vi "Battery Model Loop.vi"() -> ()   [LabVIEW 2014]
uses:
  Current Voltage Sample.ctl
  <vilib>/Analysis/6fits.llb/Curve Fitting Criteria.ctl
  <vilib>/FPGAPlugInAG/sbRIO-9626/niLvFpga_Open_sbRIO-9626.vi
  Global Data.vi
  <vilib>/Utility/error.llb/Error Cluster From Error Code.vi
  <vilib>/rvi/errors/niLvFpgaAdjustHostInterfaceError.vi
  <vilib>/FPGAPlugInAG/sbRIO-9626/niLvFpga_Close_sbRIO-9626.vi
  <vilib>/rvi/interface/nirviOpenFPGA/nirviOpenFPGA.xnode
  FPGA Bitfiles/Latest.lvbitx
  <vilib>/rvi/interface/nirviReadWriteControl/nirviReadWriteControl.xnode
  <vilib>/rvi/interface/nirviCloseFPGA/nirviCloseFPGA.xnode
  NiFpgaLv.dll
  <vilib>/Analysis/NI_AALPro.lvlib
panel:
  out "IBatteryMaxTarget":dbl
  out "r^2":dbl
  out "intercept (V)":dbl
  out "slope (V / A)":dbl
  out "tICurrentAccumulated":dbl
  in  "bResetCurrentAccumulator":bool
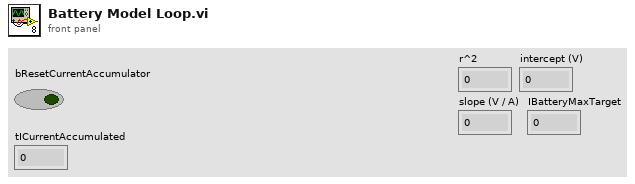
[diagram p1: front panel]
types:
  T1 = typedef "Current Voltage Sample.ctl" = cluster{"IAverage":dbl, "VCellMin":dbl, "tSampleDuration":u32}
  T2 = typedef "BMS Telemetry.ctl" = cluster{"bBMSIgnition":bool, "bBMSChargerMains":bool, "bBMSFastCharge":bool, "bBMSChargerEnabled":bool, "eBMSCarState":enum16{"Off", "On, Not Charging", "Charging", "Charging Finished", "Charging Error"}, "eBMSChargingState":enum16{"Disconnected", "Pre-charging", "Main Charging", "Balancing", "Charging Finished OK", "Charging Error"}, "tBMSChargeStage":u16, "eBMSLastChargeError":enum16{"No Error", "No Cell Communication", "No Cell Communication - Non CAN Charger", "Maximum charging stage duration expired", "Cell Communication Lost during Charge", "Cannot set balancing voltage", "Cell temps too high", "No Comms so can't determine temp", "# of Cells Mismatch", "Cells Overvoltage", "Cell Protection Event occured."}, "NBMSNumCells":u8, "bBMSUnderVProtection":bool, "bBMSOverVProtection":bool, "bBMSOverTProtection":bool, "bBMSLeakageProtection":bool, "bBMSNoCellCommsError":bool, "bBMSLowVReduction":bool, "bBMSHighTReduction":bool, "VCellMin":dbl, "VCellMax":dbl, "VCellMean":dbl, "VTotal":dbl, "TCellMin":dbl, "TCellMax":dbl, "TCellMean":dbl, "VCells":cluster{"[51]":dbl, "[52]":dbl, "[53]":dbl, "[54]":dbl, "[55]":dbl, "[56]":dbl, "[57]":dbl, "[58]":dbl, "[59]":dbl, "[60]":dbl, "[61]":dbl, "[62]":dbl, "[63]":dbl, "[64]":dbl, "[65]":dbl, "[66]":dbl, "[67]":dbl, "[34]":dbl, "[35]":dbl, "[36]":dbl, "[37]":dbl, "[38]":dbl, "[39]":dbl, "[40]":dbl, "[41]":dbl, "[42]":dbl, "[43]":dbl, "[44]":dbl, "[45]":dbl, "[46]":dbl, "[47]":dbl, "[48]":dbl, "[49]":dbl, "[50]":dbl, "[17]":dbl, "[18]":dbl, "[19]":dbl, "[20]":dbl, "[21]":dbl, "[22]":dbl, "[23]":dbl, "[24]":dbl, "[25]":dbl, "[26]":dbl, "[27]":dbl, "[28]":dbl, "[29]":dbl, "[30]":dbl, "[31]":dbl, "[32]":dbl, "[33]":dbl, "[0]":dbl, "[1]":dbl, "[2]":dbl, "[3]":dbl, "[4]":dbl, "[5]":dbl, "[6]":dbl, "[7]":dbl, "[8]":dbl, "[9]":dbl, "[10]":dbl, "[11]":dbl, "[12]":dbl, "[13]":dbl, "[14]":dbl, "[15]":dbl, "[16]":dbl}, "TCells":cluster{"[55]":dbl, "[56]":dbl, "[57]":dbl, "[58]":dbl, "[59]":dbl, "[60]":dbl, "[61]":dbl, "[62]":dbl, "[63]":dbl, "[64]":dbl, "[65]":dbl, "[66]":dbl, "[67]":dbl, "[68]":dbl, "[69]":dbl, "[70]":dbl, "[17]":dbl, "[38]":dbl, "[39]":dbl, "[40]":dbl, "[41]":dbl, "[42]":dbl, "[43]":dbl, "[44]":dbl, "[45]":dbl, "[46]":dbl, "[47]":dbl, "[48]":dbl, "[49]":dbl, "[50]":dbl, "[51]":dbl, "[52]":dbl, "[53]":dbl, "[54]":dbl, "[21]":dbl, "[22]":dbl, "[23]":dbl, "[24]":dbl, "[25]":dbl, "[26]":dbl, "[27]":dbl, "[28]":dbl, "[29]":dbl, "[30]":dbl, "[31]":dbl, "[32]":dbl, "[33]":dbl, "[34]":dbl, "[35]":dbl, "[36]":dbl, "[37]":dbl, "[0]":dbl, "[1]":dbl, "[2]":dbl, "[3]":dbl, "[4]":dbl, "[5]":dbl, "[6]":dbl, "[7]":dbl, "[8]":dbl, "[9]":dbl, "[10]":dbl, "[11]":dbl, "[12]":dbl, "[13]":dbl, "[14]":dbl, "[15]":dbl, "[16]":dbl}, "bChargerConnected":bool, "VChargerSetpoint":dbl, "IChargerSetpoint":dbl, "VChargerActual":dbl, "IChargerActual":dbl, "BCells":cluster{"[51]":dbl, "[52]":dbl, "[53]":dbl, "[54]":dbl, "[55]":dbl, "[56]":dbl, "[57]":dbl, "[58]":dbl, "[59]":dbl, "[60]":dbl, "[61]":dbl, "[62]":dbl, "[63]":dbl, "[64]":dbl, "[65]":dbl, "[66]":dbl, "[67]":dbl, "[34]":dbl, "[35]":dbl, "[36]":dbl, "[37]":dbl, "[38]":dbl, "[39]":dbl, "[40]":dbl, "[41]":dbl, "[42]":dbl, "[43]":dbl, "[44]":dbl, "[45]":dbl, "[46]":dbl, "[47]":dbl, "[48]":dbl, "[49]":dbl, "[50]":dbl, "[17]":dbl, "[18]":dbl, "[19]":dbl, "[20]":dbl, "[21]":dbl, "[22]":dbl, "[23]":dbl, "[24]":dbl, "[25]":dbl, "[26]":dbl, "[27]":dbl, "[28]":dbl, "[29]":dbl, "[30]":dbl, "[31]":dbl, "[32]":dbl, "[33]":dbl, "[0]":dbl, "[1]":dbl, "[2]":dbl, "[3]":dbl, "[4]":dbl, "[5]":dbl, "[6]":dbl, "[7]":dbl, "[8]":dbl, "[9]":dbl, "[10]":dbl, "[11]":dbl, "[12]":dbl, "[13]":dbl, "[14]":dbl, "[15]":dbl, "[16]":dbl}, "bNewVCellMinSample":bool}
  T3 = typedef "NI_AALPro.lvlib/Curve Fitting Criteria.ctl" = u16
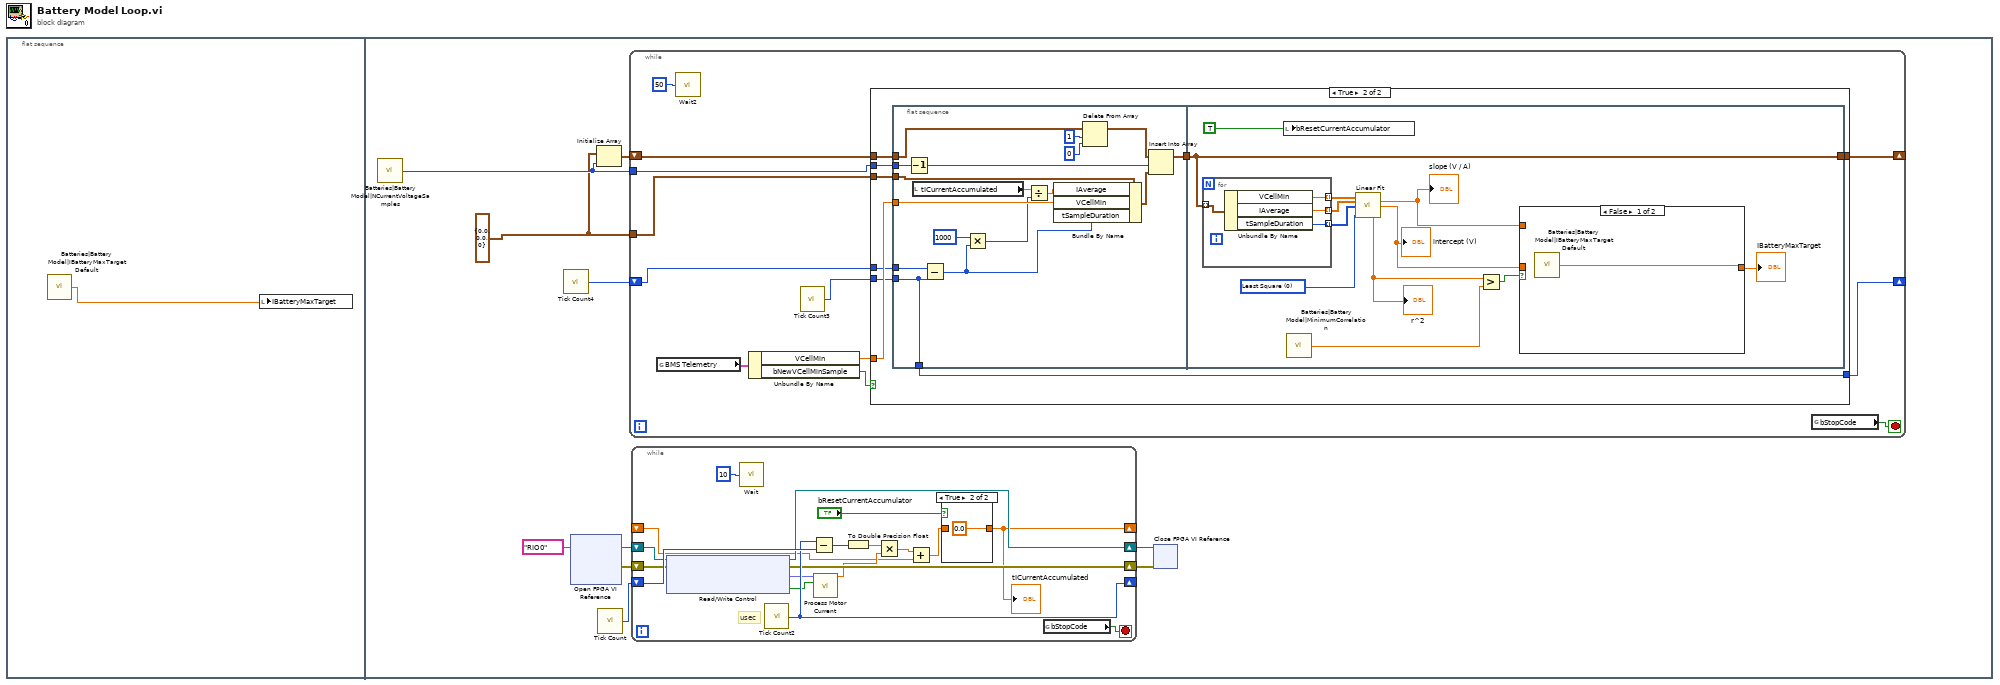
[diagram p0: block diagram]
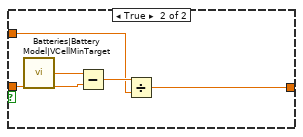
[diagram p4: hidden frame]
diagram:
  n1 = flat-sequence {
    frame #0 {
      n2 = call "Batteries|Battery Model|IBatteryMaxTargetDefault"() -> ("Value"=w1:sgl)
      n3 = local write "IBatteryMaxTarget"(w1) -> ()
    }
    frame #1 {
      w3 = T1 {"IAverage"=0.0, "VCellMin"=0.0, "tSampleDuration"=0} ("Current Voltage Sample")
      n4 = call "Batteries|Battery Model|NCurrentVoltageSamples"() -> ("Value"=w10:i32)
      n5 = call "Tick Count4"() -> ("Tick Count(mSec)"=w4:u32)
      n6 = xnode "Open FPGA VI Reference"("resource name"=tag "RIO0") -> ("FPGA VI Reference Out"=w8:refnum<k20>, "error out"=w7:errorcluster)  [unwired: 1 in]
      n7 = Initialize Array(w3, w10) -> (w11:T1[])
      n8 = call "Tick Count"() -> ("Tick Count(uSec)"=w9:u32)
      n9 = while {
        shift-right: [w39] -> _
        shift-left: w11 -> [w40]
        tunnel: w10 -> [w38]
        tunnel: w3 -> [w37]
        shift-right: [w32] -> _
        shift-left: w4 -> [w34]
        stop <- w43 stop-if-true
        n10 = global read "Global Data.vi" "BMS Telemetry"() -> (w42:T2)
        n11 = call "Wait2"("Count(mSec)"=u32 50) -> ()  [unwired: 1 out]
        n12 = Unbundle By Name(w42) -> ("VCellMin"=w36:dbl, "bNewVCellMinSample"=w41:bool)
        n13 = call "Tick Count3"() -> ("Tick Count(mSec)"=w33:u32)
        n14 = case shown="True" w41 {
          tunnel: w40 -> [w45 w54]
          tunnel: [w45 w50] -> w39
          tunnel: w38 -> [_ w53]
          tunnel: w37 -> [_ w52]
          tunnel: w36 -> [_ w51]
          tunnel: w34 -> [w44 w48]
          tunnel: w33 -> [_ w47]
          tunnel: [w44 w46] -> w32
          frame False {
          }
          frame True {
            n15 = flat-sequence {
              tunnel: w54 -> [w71]
              tunnel: w53 -> [w67]
              tunnel: w52 -> [w65]
              tunnel: w51 -> [w63]
              tunnel: [w62] -> w49
              tunnel: w48 -> [w61]
              tunnel: w47 -> [w60]
              tunnel: [w60] -> w46
              tunnel: [w82] -> w50
              tunnel: w49 -> [w82]
              frame #0 {
                n16 = Decrement(x=w67) -> (x-1=w66:i32)
                n17 = local read "tICurrentAccumulated"() -> (w58:dbl)
                n18 = Subtract(x=w61, y=w60) -> (x-y=w57:u32)
                n19 = Multiply(x=u32 1000, y=w57) -> (x*y=w55:u32)
                n20 = Divide(x=w58, y=w55) -> (x/y=w59:dbl)
                n21 = Bundle By Name(cluster=w65, "IAverage"=w59, "VCellMin"=w63, "tSampleDuration"=w57) -> (w64:T1)
                n22 = Delete From Array(array=w71, length=1, index=0) -> (array with subset deleted=w68:T1[])  [unwired: 1 out]
                n23 = Insert Into Array(array=w68, index=w66, new element=w64) -> (w62:T1[])
              }
              frame #1 {
                w78 = T3 0 items=["Least Square", "Least Absolute Residual", "Bisquare"] ("method")
                n24 = for {
                  tunnel: w82 -> [w93] mode=indexing
                  tunnel: [w92] -> w81 mode=indexing
                  tunnel: [w91] -> w80 mode=indexing
                  tunnel: [w90] -> w79 mode=indexing
                  n25 = Unbundle By Name(w93) -> ("VCellMin"=w92:dbl, "IAverage"=w91:dbl, "tSampleDuration"=w90:u32)
                }
                n26 = local write "bResetCurrentAccumulator"(TRUE ("bResetCurrentAccumulator")) -> ()
                n27 = call "Batteries|Battery Model|MinimumCorrelation"() -> ("Value"=w76:sgl)
                n28 = call <vilib>:"Linear Fit.vi"("Y"=w81, "X"=w80, "Weight"=w79, "method"=w78) -> ("slope"=w73:dbl, "intercept"=w74:dbl, "residue"=w77:dbl)  [unwired: 7 in, 2 out]
                "slope (V / A)" <- w73
                "intercept (V)" <- w74
                "r^2" <- w77
                n29 = Greater?(x=w77, y=w76) -> (0:w75:bool)
                n30 = case shown="False" w75 {
                  tunnel: w74 -> [_ w88]
                  tunnel: w73 -> [_ w86]
                  tunnel: [w84 w85] -> w72
                  frame False {
                    n31 = call "Batteries|Battery Model|IBatteryMaxTargetDefault"() -> ("Value"=w84:sgl)
                  }
                  frame True {
                    n32 = call "Batteries|Battery Model|VCellMinTarget"() -> ("Value"=w89:sgl)
                    n33 = Subtract(x=w89, y=w88) -> (x-y=w87:dbl)
                    n34 = Divide(x=w87, y=w86) -> (x/y=w85:dbl)
                  }
                }
                "IBatteryMaxTarget" <- w72
              }
            }
          }
        }
        n35 = global read "Global Data.vi" "bStopCode"() -> (w43:bool)
      }
      n36 = while {
        shift-right: [w26] -> _
        shift-left: w9 -> [w27]
        shift-right: [w21] -> w6
        shift-left: w8 -> [w25]
        shift-right: [w20] -> w5
        shift-left: w7 -> [w24]
        shift-right: [w12] -> _
        shift-left: _ -> [w15]
        stop <- w28 stop-if-true
        # "usec"
        n37 = xnode "Read/Write Control"("FPGA VI Reference In"=w25, "error in"=w24) -> ("FPGA VI Reference Out"=w21:refnum<k20>, "error out"=w20:errorcluster, "IHighCurrent"=w23:fxp<+/-,19,15>, "bHighCurrentOK"=w22:bool)
        n38 = call "Wait"("Count(mSec)"=u32 10) -> ()  [unwired: 1 out]
        n39 = call "Tick Count2"() -> ("Tick Count(uSec)"=w26:u32)
        n40 = Subtract(x=w26, y=w27) -> (x-y=w17:u32)
        n41 = call "Process Motor Current.vi"("bHighCurrentOK"=w22, "IHighCurrent"=w23) -> ("IMotor"=w19:dbl)  [unwired: 8 in, 1 out]
        n42 = To Double Precision Float(number=w17) -> (double precision float=w18:dbl)
        n43 = Multiply(x=w18, y=w19) -> (x*y=w16:dbl)
        n44 = Add(x=w16, y=w15) -> (x+y=w14:dbl)
        n45 = case shown="True" "bResetCurrentAccumulator" {
          tunnel: w14 -> [w30 _]
          tunnel: [w30 0.0] -> w12
          frame False {
          }
          frame True {
          }
        }
        "tICurrentAccumulated" <- w12
        n46 = global read "Global Data.vi" "bStopCode"() -> (w28:bool)
      }
      n47 = xnode "Close FPGA VI Reference"("FPGA VI Reference In"=w6, "error in"=w5) -> ()  [unwired: 1 out]
    }
  }
